vi "MeasureWhileChanging.vi"(8 "error in (no error)":errorcluster, 11 "ChromaAcLoad in":refnum<class "ChromaAcLoad.lvclass">) -> (0 "error out":errorcluster, 1 "MeasureWhileChangingConfigurationSettings":bool, 2 "MeasureWhileChangingOutput/LoadState":bool, 3 "AcPwrBase Out":refnum<class "AcPwrBase.lvclass">)   [LabVIEW 2018, in "AcPwrPlugins.lvlib" / "ChromaAcLoad.lvclass"]
doc: "This VI retrieves a boolean status to see if the instrument can conduct measurements while the device is changing modes or turning off and on."
uses:
  ChromaAcLoad.lvclass
  AcPwrBaseClass/AcPwrBase.lvclass
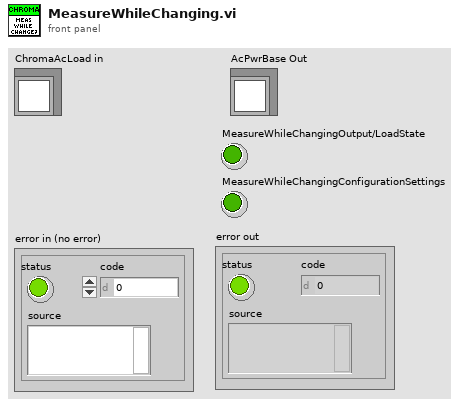
[diagram p1: front panel]
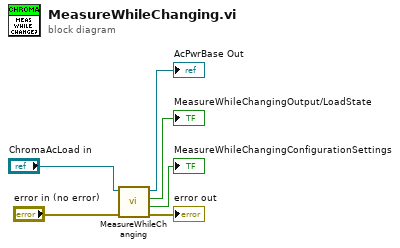
[diagram p0: block diagram]
diagram:
  n1 = call-parent "MeasureWhileChanging.vi"("error in (no error)"="error in (no error)", "AcPwrBase in"="ChromaAcLoad in") -> ("error out"=→"error out":errorcluster, "MeasureWhileChangingConfigurationSettings"=→"MeasureWhileChangingConfigurationSettings":bool, "MeasureWhileChangingOutput/LoadState"=→"MeasureWhileChangingOutput/LoadState":bool, "AcPwrBase Out"=→"AcPwrBase Out":refnum<class "AcPwrBase.lvclass">)  [unwired: 6 in]
